vi "TDC_generateTimestamps.vi"(0 "Distribution":i32(ring) items=["Flat", "Normal", "None"], 1 "Parameters":dbl[](array[numeric]), 2 "Count":i32, 3 "Error In":errorcluster) -> (10 "Error Out":errorcluster)   [LabVIEW 2011]
uses:
  tdcbase.dll
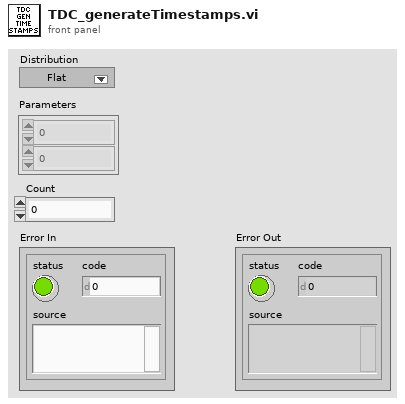
[diagram p1: front panel]
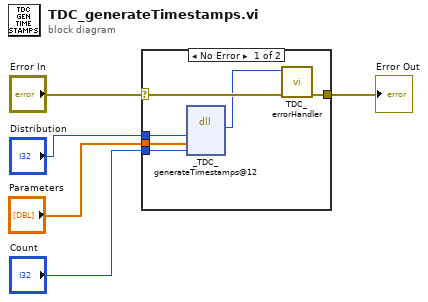
[diagram p0: block diagram]
diagram:
  n1 = case shown="No Error" "Error In" {
    selector: "Error In" -> [w11 w12]
    tunnel: [w10 w12] -> w4
    tunnel: "Distribution" -> [w8 _]
    tunnel: "Parameters" -> [w7 _]
    tunnel: "Count" -> [w6 _]
    frame No Error {
      n2 = dll-call lib="X:/tdcbase.dll" fn="_TDC_generateTimestamps@12"("type"=w8, "parameters"=w7, "count"=w6) -> ("return type"=w9:i32)  [unwired: 6 in, 2 out]
      n3 = call "TDC_errorHandler.vi"("Error In"=w11, "TDC Return Code"=w9) -> ("Error Out"=w10:errorcluster)  [unwired: 9 in]
    }
    frame Error {
    }
  }
  "Error Out" <- w4
